vi "RT_Gravitational_Force_in_DLR_Body_Reference_System (SubVI).vi"(9 "Rotation":T1, 11 "FG_d":dbl[](array[numeric])) -> (3 "FG_b":dbl[](array[numeric]))   [LabVIEW 2017]
uses:
  <vilib>/Analysis/baseanly.llb/Real A x B.vi
  <vilib>/Analysis/Matrix/Numeric/Conversions/Array To Matrix - RA.vi
  <vilib>/Analysis/Matrix/Numeric/Conversions/Array To Matrix - RA2.vi
  <vilib>/Analysis/Matrix/Numeric/Conversions/Matrix To Array - RM.vi
  <vilib>/Analysis/NI_AALBase.lvlib
  <vilib>/Analysis/Matrix/NI_Matrix.lvlib
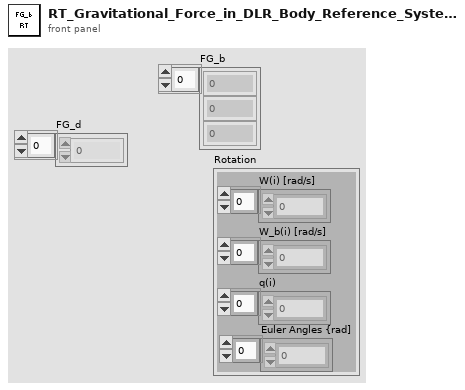
[diagram p1: front panel]
types:
  T1 = cluster{"W(i) [rad/s]":dbl[], "W_b(i) [rad/s]":dbl[], "q(i)":dbl[], "Euler Angles {rad]":dbl[]}
  T2 = typedef "NI_Matrix.lvlib/RealMatrix.ctl" = dbl[][]
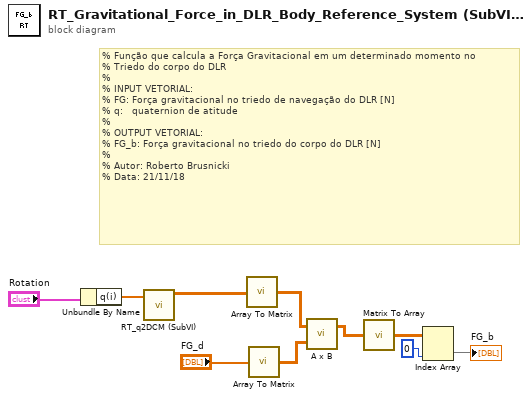
[diagram p0: block diagram]
diagram:
  # "% Função que calcula a Força Gravitacional em um determinado momento no \n% Triedo do corpo do DLR\n%\n% INPUT VETORIAL: \n% FG: Força gravitacional no triedo de navegação do DLR [N]\n% q:   quaternion de atitude   \n%\n% OUTPUT VETORIAL:\n% FG_b: Força gravitacional no triedo do corpo do DLR [N]\n%\n% Autor: Roberto Brusnicki\n% Data: 21/11/18"
  n1 = Unbundle By Name("Rotation") -> ("q(i)"=w3:dbl[])
  n2 = call "RT_q2DCM (SubVI).vi"("Quaternion"=w3) -> ("DCM"=w2:dbl[][])  [unwired: 10 in]
  n3 = call-poly <vilib>:"Array To Matrix.vi"("Real 2D Array"=w2) -> ("Real Matrix"=w8:T2)
  n4 = call-poly <vilib>:"Array To Matrix.vi"("Real 1D Array"="FG_d") -> ("Real Matrix (Column Vector)"=w5:T2)
  n5 = call-poly <vilib>:"A x B.vi"("B"=w5, "A"=w8) -> ("A x B"=w10:T2)  [unwired: 1 out]
  n6 = call-poly <vilib>:"Matrix To Array.vi"("Real Matrix"=w10) -> ("Real 2D Array"=w6:dbl[][])
  n7 = Index Array(array=w6, index (col)=0 ("index (row)")) -> (element=→"FG_b":dbl[])  [unwired: 1 in]
